vi "Open_first_camera.vi"(8 "error in":errorcluster) -> (0 "error out":errorcluster, 3 "camera handle out":u64)   [LabVIEW 2014, in "PICam.lvlib"]
doc: "Picam_OpenFirstCamera() opens the first available camera, and returns a handle to the\ncamera."
uses:
  PICam.lvlib
  Program Files/Princeton Instruments/PICam/Runtime/Picam32.dll
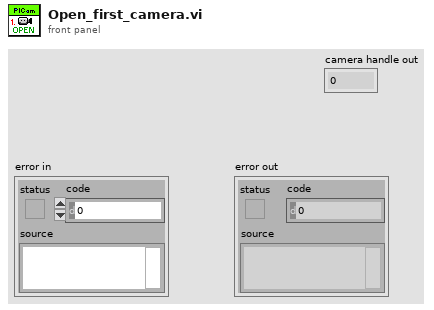
[diagram p1: front panel]
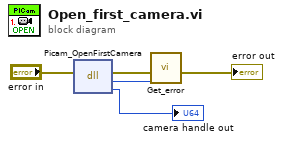
[diagram p0: block diagram]
diagram:
  n1 = dll-call lib="C:/Program Files/Princeton Instruments/PICam/Runtime/Picam32.dll" fn="Picam_OpenFirstCamera"(error in="error in") -> (error out=w3:errorcluster, "return type"=w2:i32, "camera handler"=→"camera handle out":u64)  [unwired: 3 in, 1 out]
  n2 = call "Get_error.vi"("PICam_Error"=w2, "error in (no error)"=w3) -> ("error out"=→"error out":errorcluster)  [unwired: 9 in]
